vi "SignProvider.vi"() -> ()   [LabVIEW 2018]
uses:
  <vilib>/Utility/config.llb/NI_LVConfig.lvlib
  <vilib>/Utility/config.llb/Read Key (String).vi
  Program Files (x86)/National Instruments/LabVIEW 2020/user.lib/_OpenG.lib/md5/md5.llb/MD5 Message Digest (Hexadecimal String)__ogtk.vi
  <vilib>/Utility/config.llb/Write Key (String).vi
panel:
  out "Signature":string
  in  "File Path":path
  # "Add the signature to the ini file"
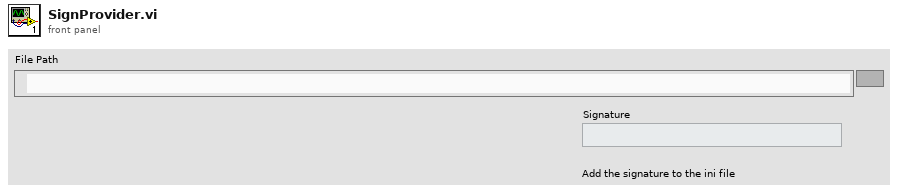
[diagram p1: front panel]
types:
  T1 = typedef "NI_LVConfig.lvlib/Config Data RefNum.ctl" = refnum<k1>
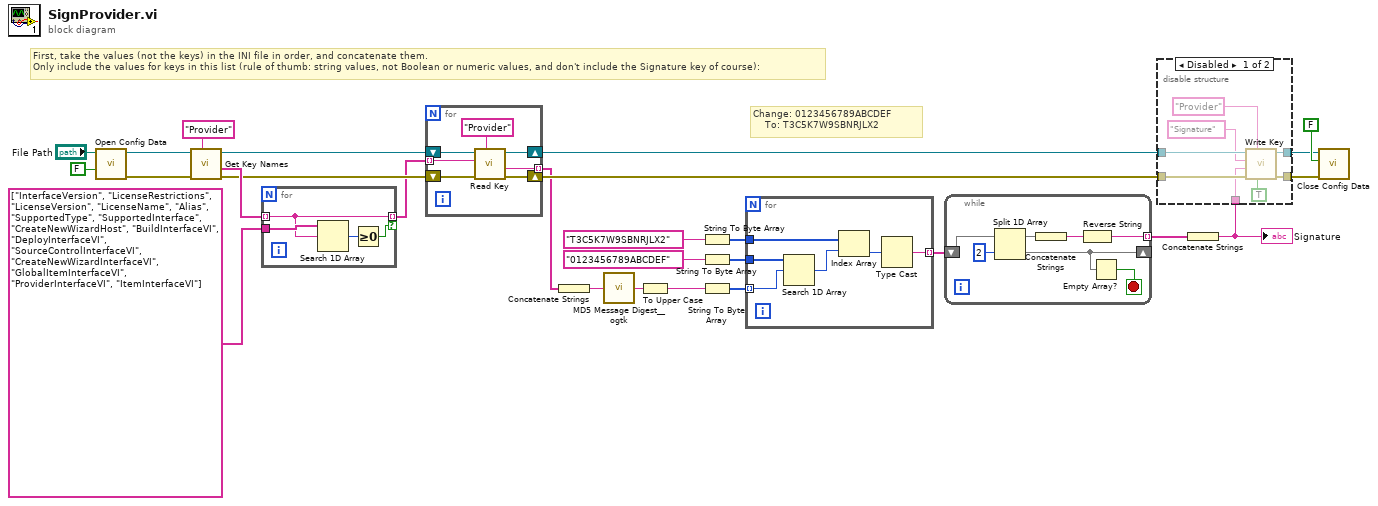
[diagram p0: block diagram]
diagram:
  # "Change: 0123456789ABCDEF\n    To: T3C5K7W9SBNRJLX2"
  # "First, take the values (not the keys) in the INI file in order, and concatenate them. \nOnly include the values for keys in this list (rule of thumb: string values, not Boolean or numeric values, and don't include the Signature key of course):"
  n1 = call <vilib>:"Open Config Data.vi"("create file if necessary (T)"=FALSE, "configuration file path"="File Path") -> ("error out"=w22:errorcluster, "refnum"=w24:T1)  [unwired: 7 in, 1 out]
  n2 = call <vilib>:"Get Key Names.vi"("section"="Provider", "error in (no error)"=w22, "refnum"=w24) -> ("error out"=w18:errorcluster, "key names"=w21:string[], "refnum out"=w19:T1)  [unwired: 5 in, 1 out]
  n3 = for {
    tunnel: w21 -> [w29] mode=indexing
    tunnel: string[] ["InterfaceVersion", "LicenseRestrictions", "LicenseVersion", "LicenseName", "Alias", "SupportedType", "SupportedInterface", "CreateNewWizardHost", "BuildInterfaceVI", "DeployInterfaceVI", "SourceControlInterfaceVI", "CreateNewWizardInterfaceVI", "GlobalItemInterfaceVI", "ProviderInterfaceVI", "ItemInterfaceVI"] -> [w30]
    tunnel: [w29] -> w16 mode=indexing if=w31
    n4 = Search 1D Array(1D array=w30, element=w29) -> (index of element=w28:i32)  [unwired: 1 in]
    n5 = Greater Or Equal To 0?(x=w28) -> (x >= 0?=w31:bool)
  }
  n6 = for {
    shift-right: [w35] -> w7
    shift-left: w19 -> [w38]
    shift-right: [w36] -> w17
    shift-left: w18 -> [w37]
    tunnel: w16 -> [w33] mode=indexing
    tunnel: [w32] -> w15 mode=indexing
    n7 = call-poly <vilib>:"Read Key.vi"("section"="Provider", "error in (no error)"=w37, "key"=w33, "refnum"=w38) -> ("error out"=w36:errorcluster, "value"=w32:string, "refnum out"=w35:T1)  [unwired: 4 in, 1 out]
  }
  n8 = Concatenate Strings(w15) -> (w14:string)
  n9 = call-poly "MD5 Message Digest__ogtk.vi"("Message"=w14) -> ("MD5 Message Digest"=w13:string)
  n10 = To Upper Case(1:w13) -> (0:w11:string)
  n11 = String To Byte Array(string="T3C5K7W9SBNRJLX2") -> (unsigned byte array=w2:u8[])
  n12 = String To Byte Array(string="0123456789ABCDEF") -> (unsigned byte array=w1:u8[])
  n13 = String To Byte Array(string=w11) -> (unsigned byte array=w12:u8[])
  n14 = for {
    tunnel: w12 -> [w40] mode=indexing
    tunnel: [w43] -> w10 mode=indexing
    tunnel: w2 -> [w42]
    tunnel: w1 -> [w41]
    n15 = Search 1D Array(1D array=w41, element=w40) -> (index of element=w39:i32)  [unwired: 1 in]
    n16 = Index Array(array=w42, index=w39) -> (element=w44:u8)
    n17 = Type Cast(x=w44) -> (*(type *) &x=w43:string)  [unwired: 1 in]
  }
  n18 = while {
    shift-right: [w48] -> _
    shift-left: w10 -> [w51]
    tunnel: [w45] -> w9 mode=indexing
    stop <- w47 stop-if-true
    n19 = Split 1D Array(array=w51, index=2) -> (first subarray=w49:string[], second subarray=w48:string[])
    n20 = Concatenate Strings(w49) -> (w46:string)
    n21 = Reverse String(1:w46) -> (0:w45:string)
    n22 = Empty Array?(array=w48) -> (empty?=w47:bool)
  }
  n23 = Concatenate Strings(w9) -> (w5:string)
  "Signature" <- w5
  n24 = disable-structure shown="Disabled" {
    disable-tunnel: w17 -> [w59 w60]
    disable-tunnel: [w58 w60] -> w8
    disable-tunnel: w7 -> [w57 w61]
    disable-tunnel: [w56 w61] -> w6
    disable-tunnel: w5 -> [w53 _]
    frame Disabled {
      n25 = call-poly <vilib>:"Write Key.vi"("write raw string? (F)"=TRUE, "section"="Provider", "error in (no error)"=w59, "value"=w53, "key"="Signature", "refnum"=w57) -> ("error out"=w58:errorcluster, "refnum out"=w56:T1)  [unwired: 3 in, 1 out]
    }
    frame Enabled {
    }
  }
  n26 = call <vilib>:"Close Config Data.vi"("error in (no error)"=w8, "write file if changed (T)"=FALSE, "refnum"=w6) -> ()  [unwired: 7 in, 2 out]
